vi "Car Wash.vi"() -> ()   [LabVIEW 2021]
doc: "car wash by Jeremy"
uses:
  Controls/Car Wash Indicators.ctl
  Controls/Wash Options.ctl
  Controls/states.ctl
panel:
  in  "Start":bool
  out "Elapsed Time":dbl format="%0.2f"
  in  "stop":bool
  out "Wash Entry":bool
  in  "Wash Options":T1
  in  "Car Position Slider":u8(slide) max=3 scale=0.0..4.0
  out "Car Wash Indicators":T2
  # "Entry Console"
  # "Car Wash Display"
  # "Car Position Simulation"
  # "Pre-Soak\nH-P Wash\nL-P Wax\nSpot Free Rinse"
  # "Underbody Wash\nBug Remover"
  # "Tire Shine\nAir Dry"
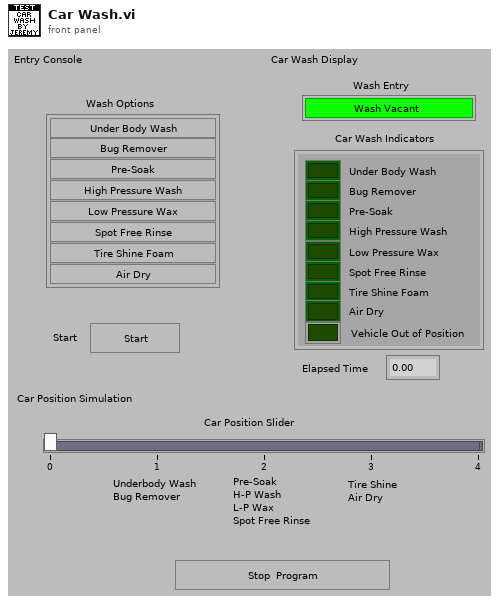
[diagram p1: front panel]
types:
  T1 = typedef "Wash Options.ctl" = cluster{"Underbody Wash":bool, "Bug Remover":bool, "Pre-Soak":bool, "High Pressure Wash":bool, "Low Pressure Wax":bool, "Spot Free Rinse":bool, "Tire Shine Foam":bool, "Air Dry":bool}
  T2 = typedef "Car Wash Indicators.ctl" = cluster{"Under Body Wash":bool, "Bug Remover":bool, "Pre-Soak":bool, "High Pressure Wash":bool, "Low Pressure Wax":bool, "Spot Free Rinse":bool, "Tire Shine Foam":bool, "Air Dry":bool, "Vehicle Out of Position":bool}
  T3 = typedef "states.ctl" = enum16{"Init", "Select Wash Options", "Configure Options", "Under Body Wash", "Bug Remover", "Pre-Soak", "High Pressure Wash", "Low Pressure Wax", "Spot Free Rinse", "Tire Shine Foam", "Air Dry", "Skip", "Exit", "Stop"}
  T4 = enum8{"Enabled", "Disabled", "Disabled and Grayed Out"}
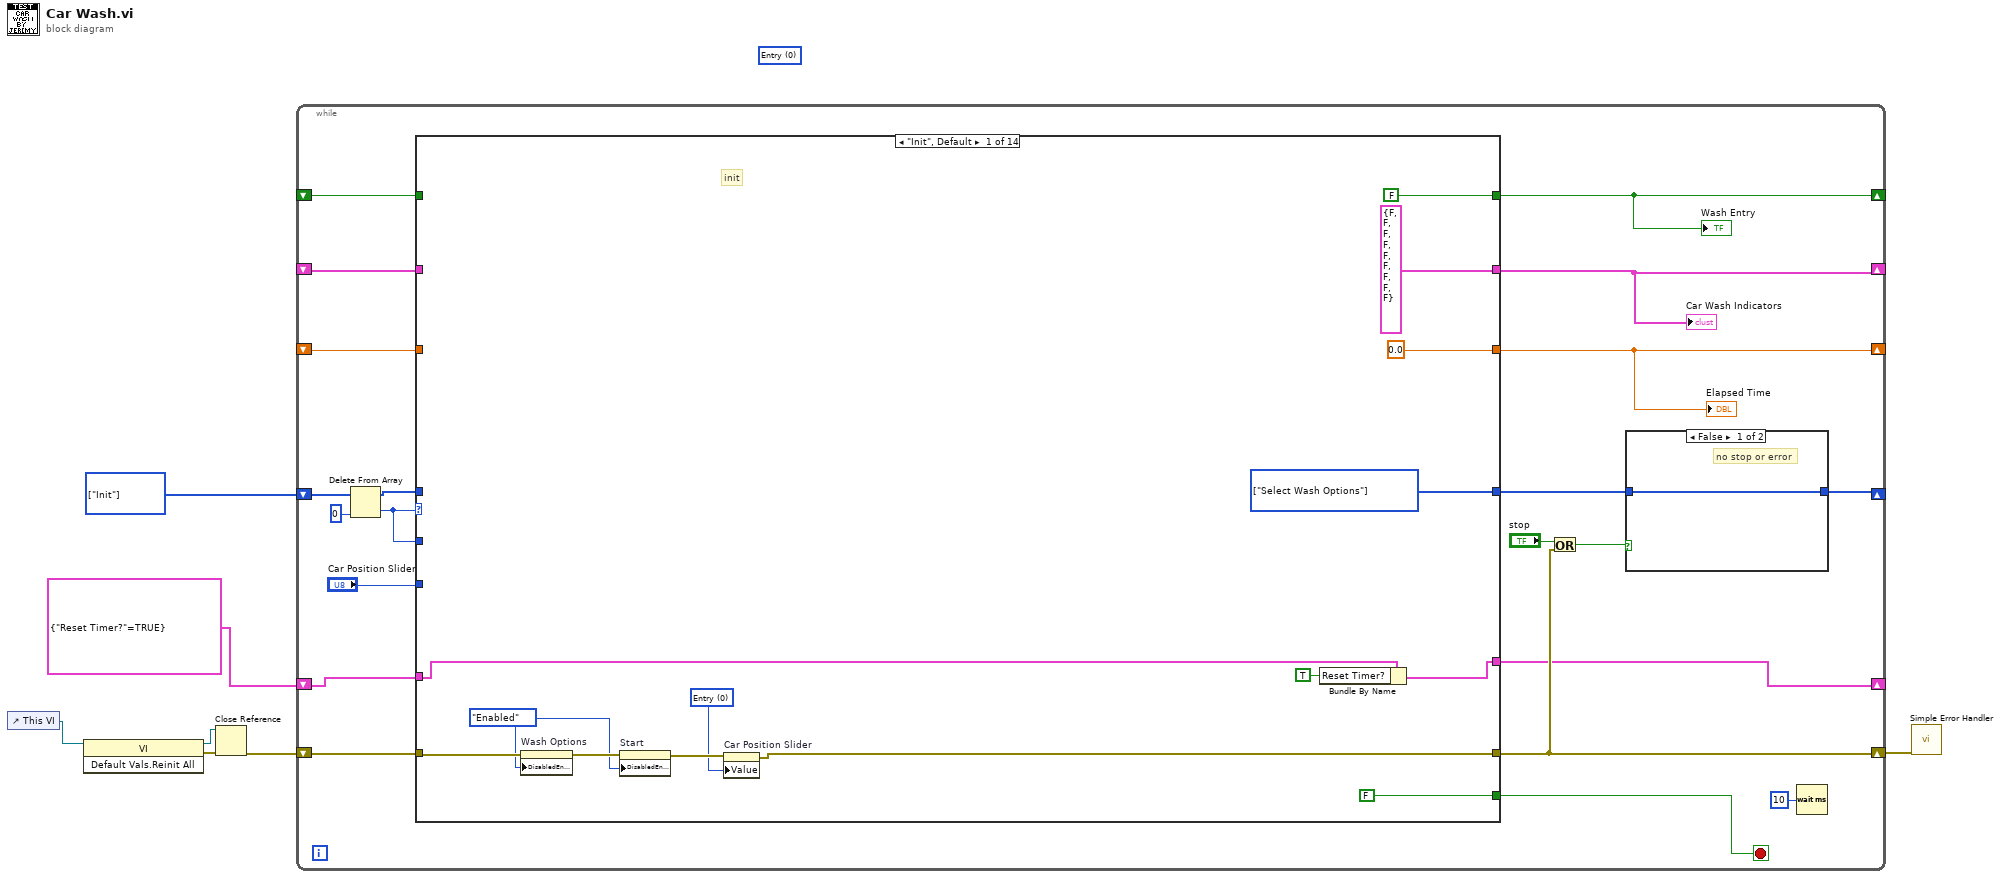
[diagram p0: block diagram]
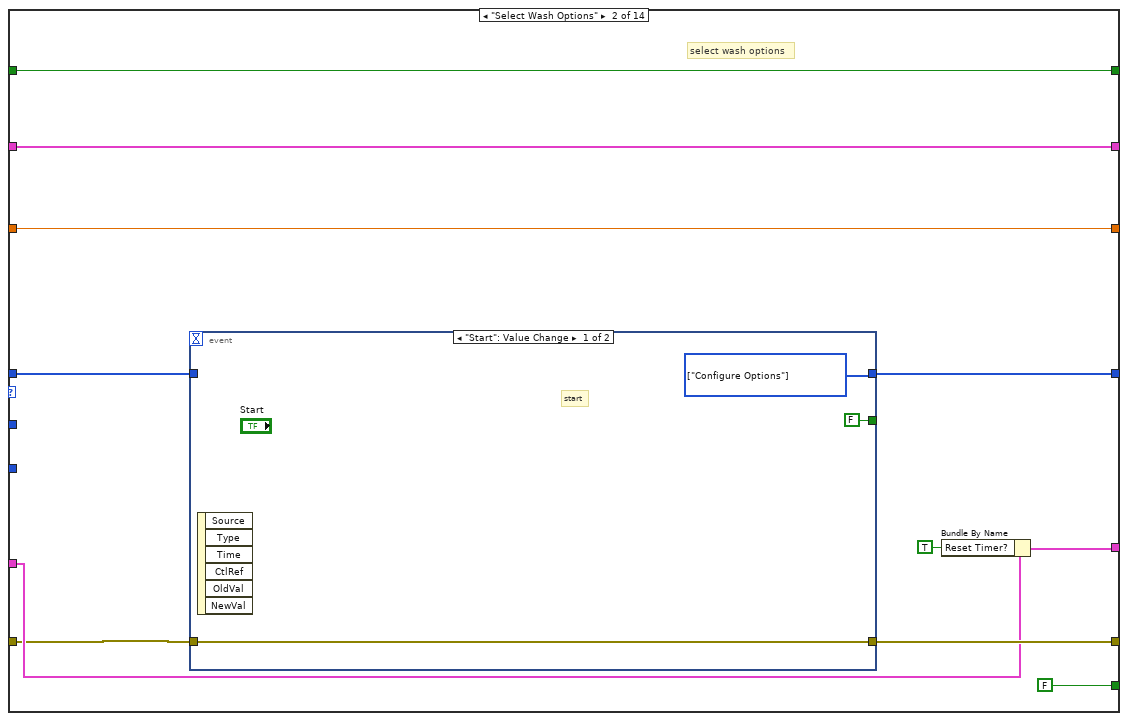
[diagram p2: hidden frame]
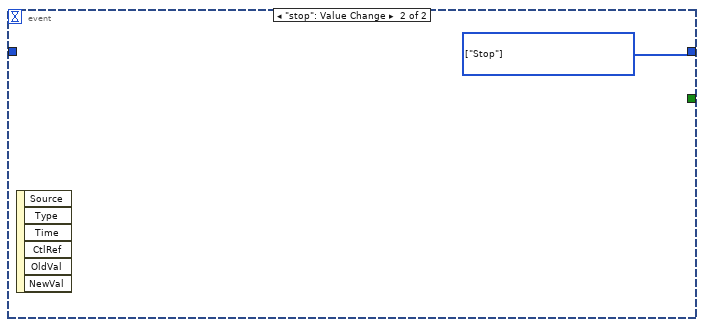
[diagram p3: hidden frame]
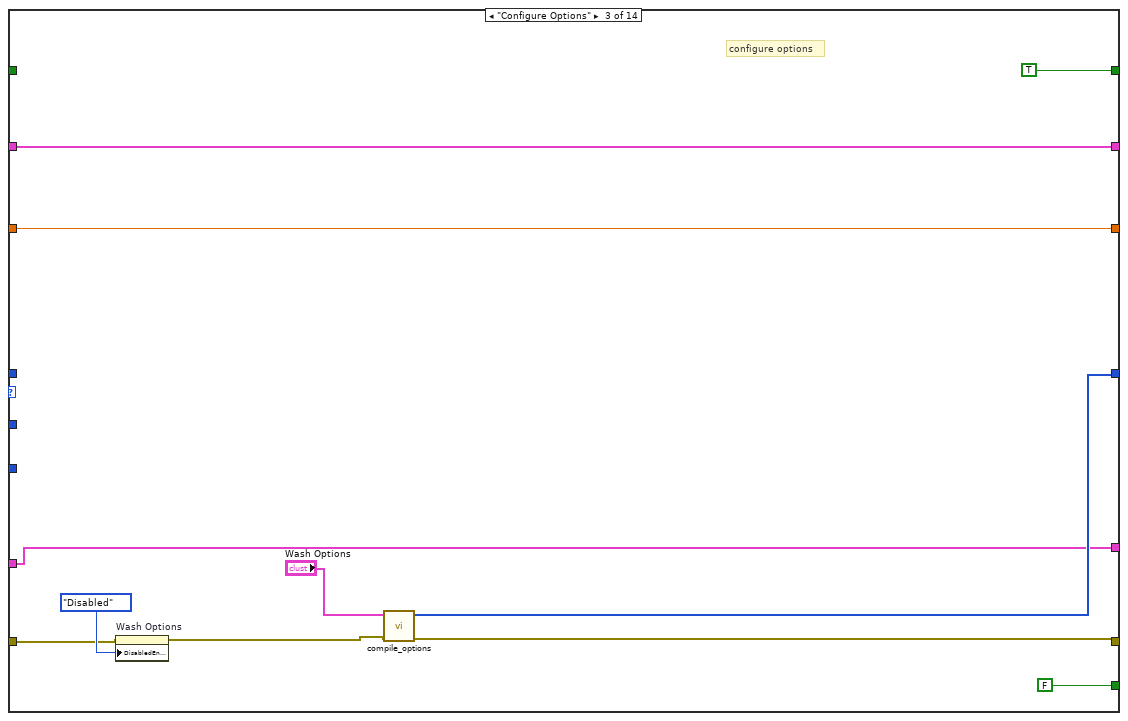
[diagram p4: hidden frame]
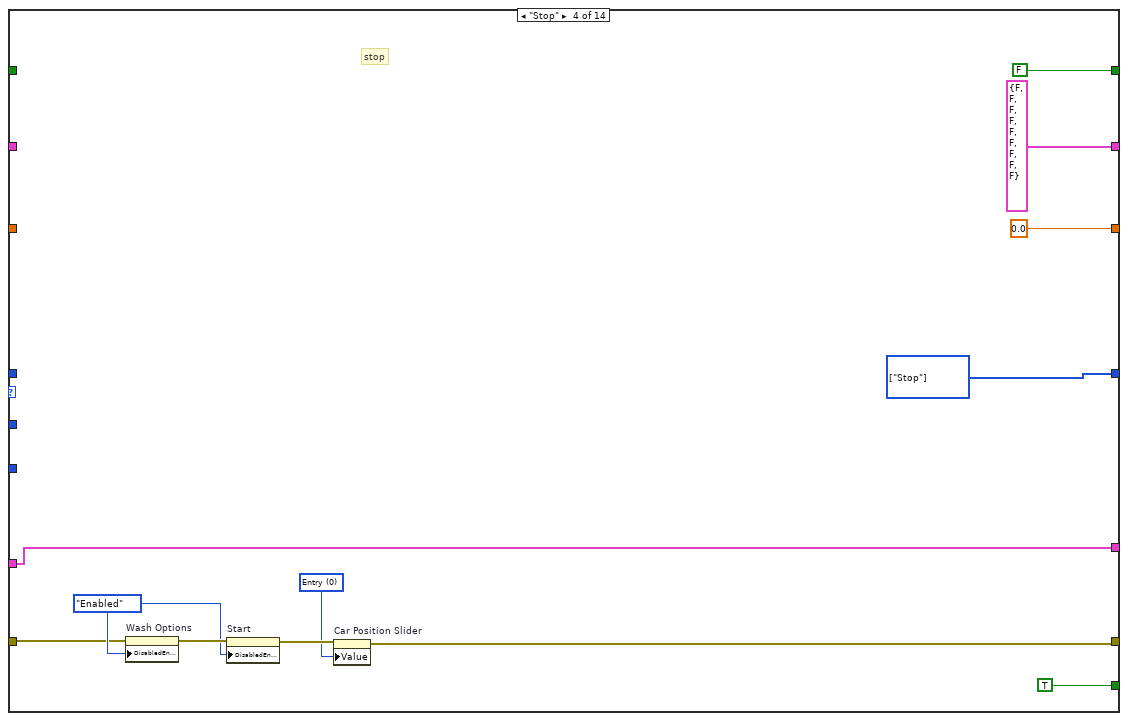
[diagram p5: hidden frame]
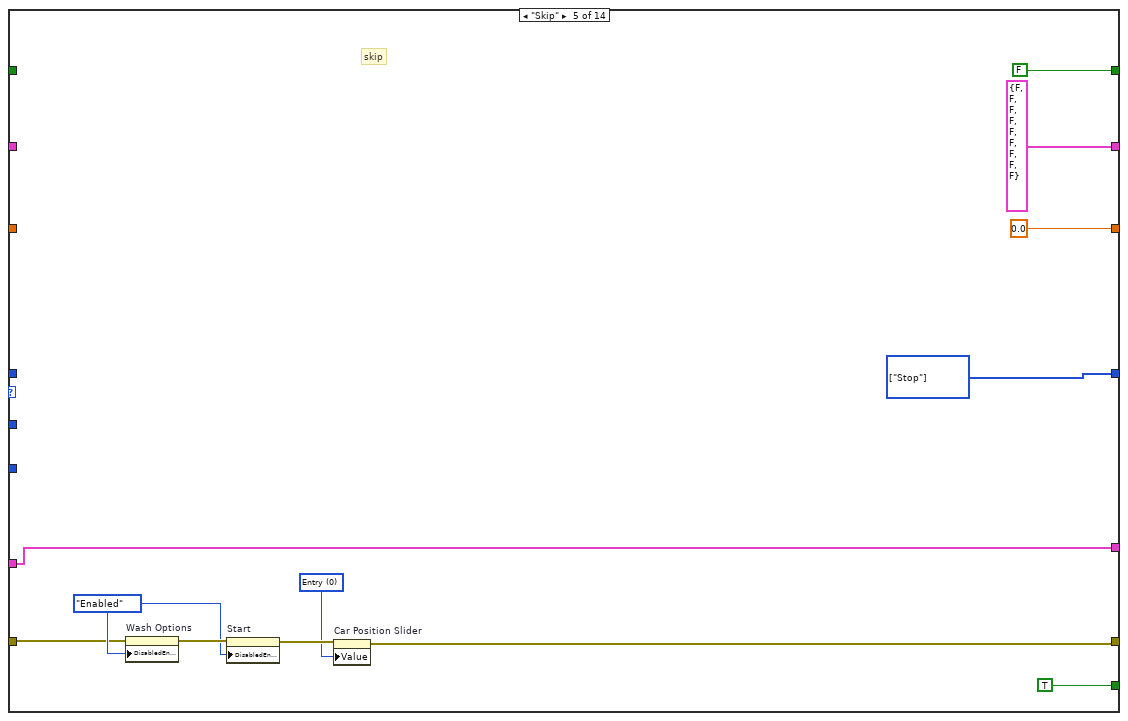
[diagram p6: hidden frame]
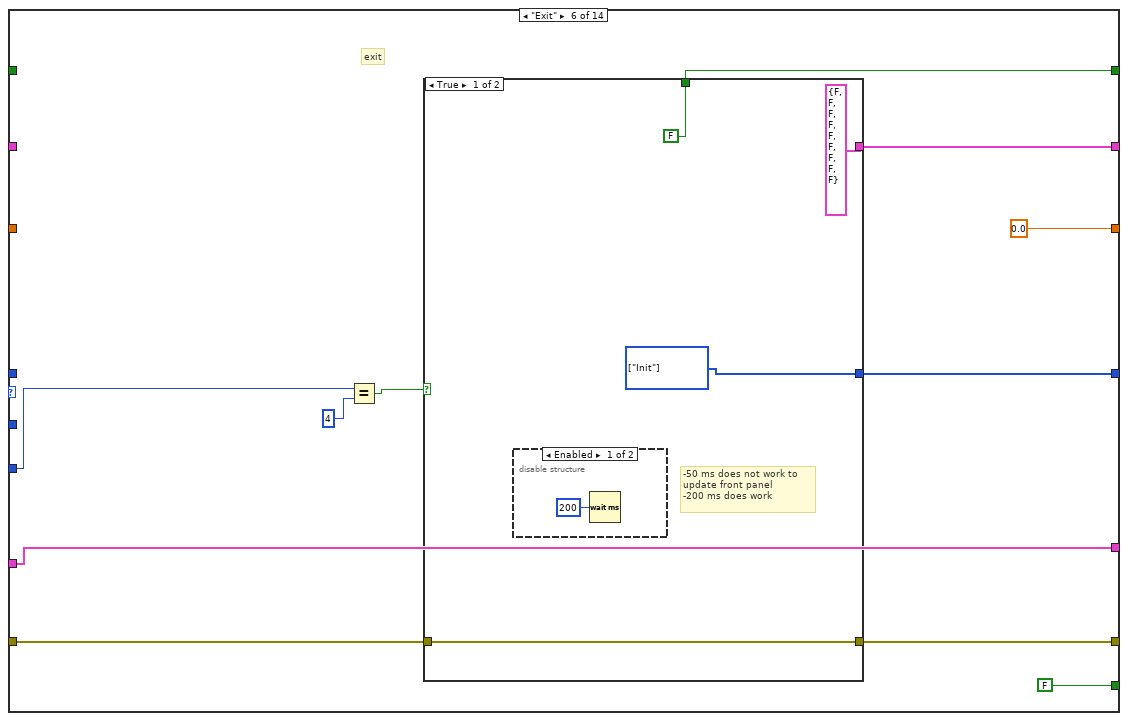
[diagram p7: hidden frame]
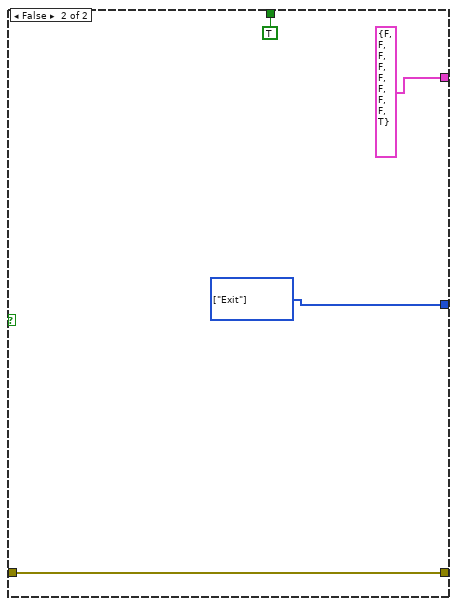
[diagram p9: hidden frame]
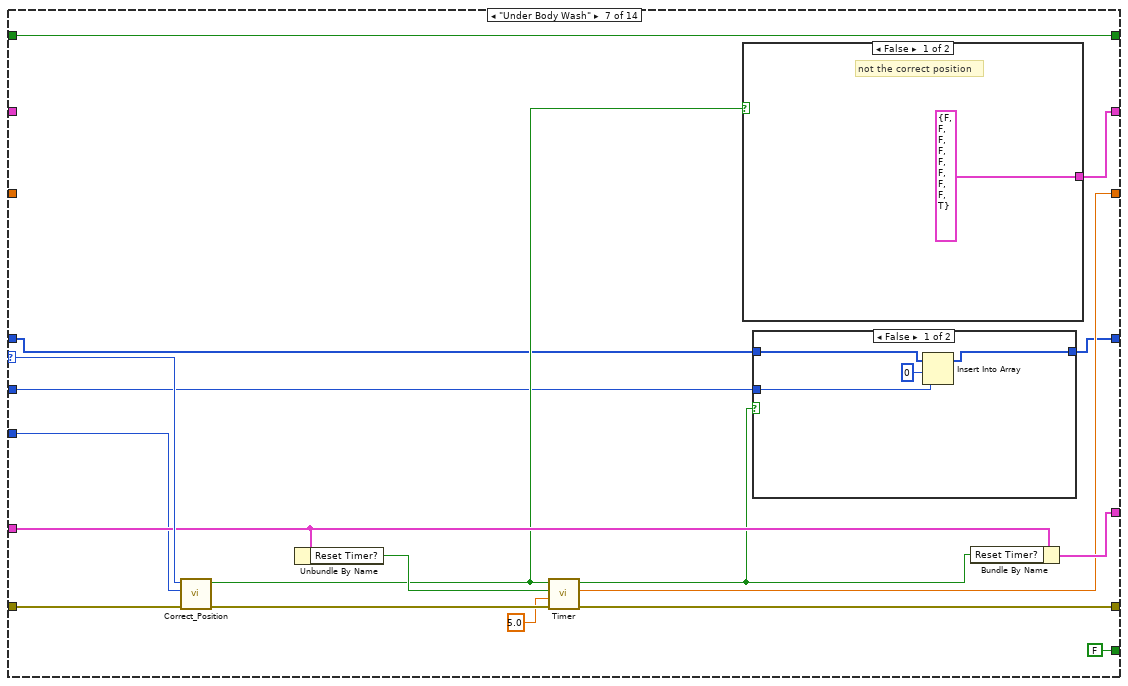
[diagram p10: hidden frame]
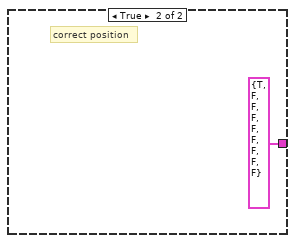
[diagram p12: hidden frame]
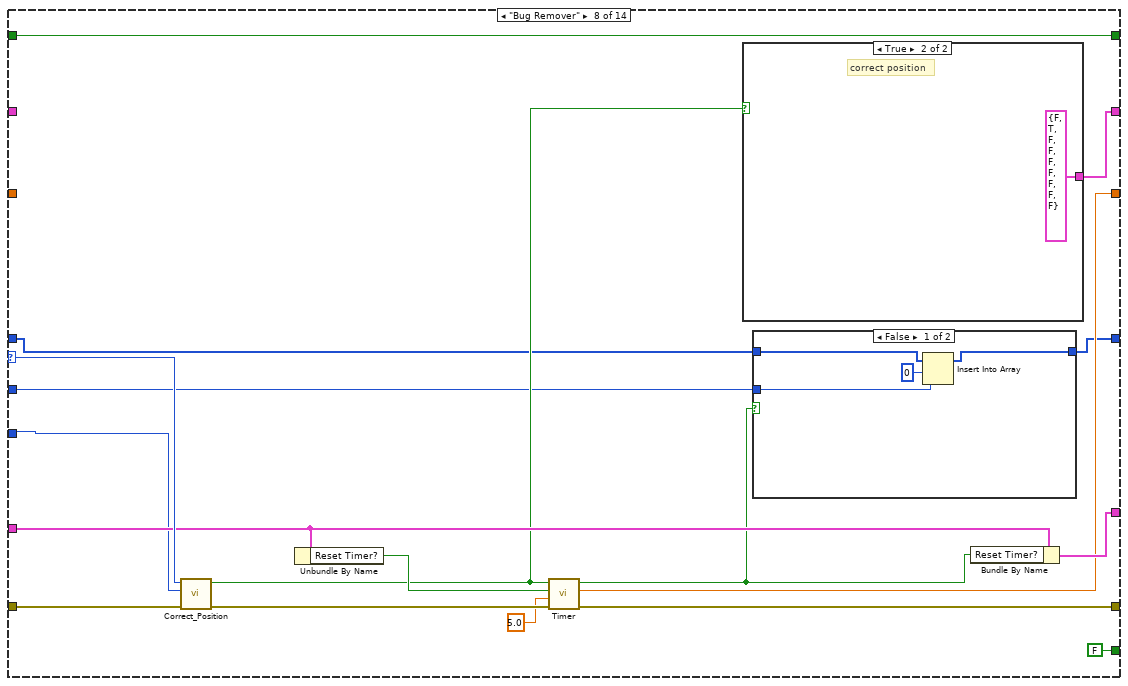
[diagram p13: hidden frame]
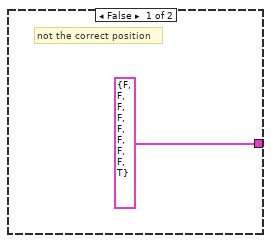
[diagram p15: hidden frame]
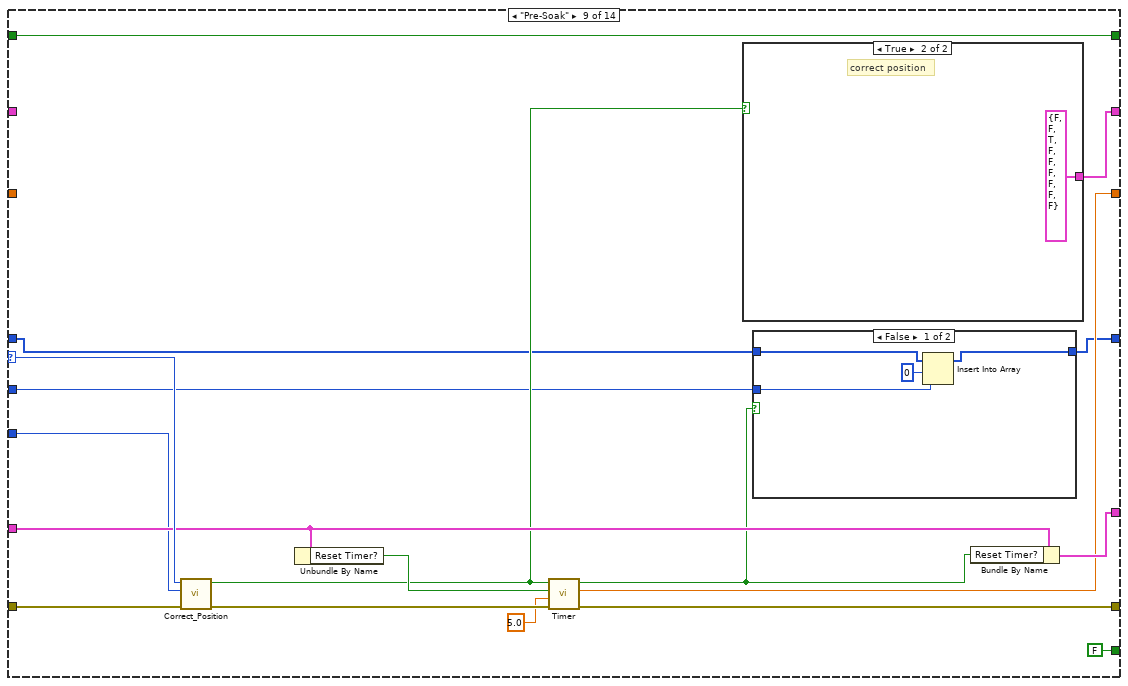
[diagram p16: hidden frame]
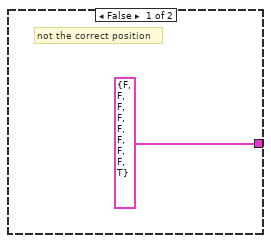
[diagram p18: hidden frame]
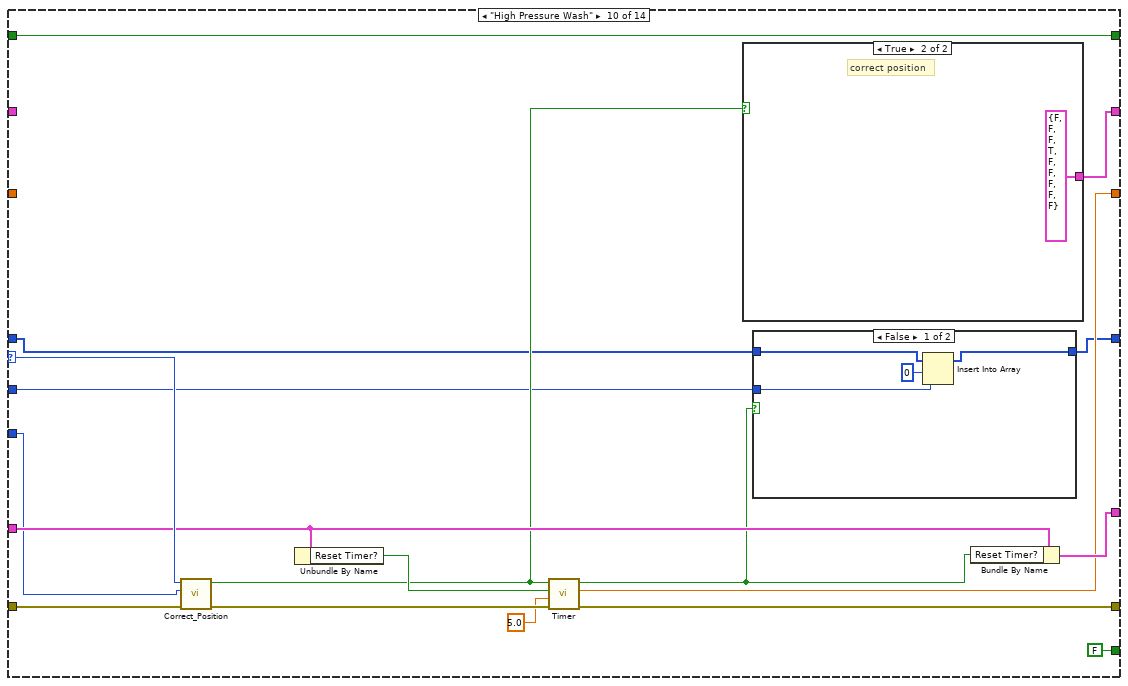
[diagram p19: hidden frame]
diagram:
  (unwired) u8 0 items=["Entry", "Station 1", "Station 2", "Station 3", "Exit"] ("Car Position Slider")
  w4 = T3[] [enum."Init"] items=["Init", "Select Wash Options", "Configure Options", "Under Body Wash", "Bug Remover", "Pre-Soak", "High Pressure Wash", "Low Pressure Wax", "Spot Free Rinse", "Tire Shine Foam", "Air Dry", "Skip", "Exit", "Stop"]
  n1 = control-ref of="This VI"() -> (w7:refnum<vi>)
  n2 = invoke class="VI" method="Default Vals.Reinit All"(reference=w7) -> (reference out=w5:refnum<vi>, error out=w6:errorcluster)  [unwired: 2 in, 1 out]
  n3 = Close Reference(reference=w5, error in (no error)=w6) -> (error out=w1:errorcluster)
  n4 = while {
    shift-right: [w17] -> w2
    shift-left: w1 -> [w9]
    shift-right: [w19] -> _
    shift-left: w4 -> [w28]
    shift-right: [w21] -> _
    shift-left: _ -> [w24]
    shift-right: [w20] -> _
    shift-left: _ -> [w25]
    shift-right: [w22] -> _
    shift-left: _ -> [w23]
    shift-right: [w13] -> _
    shift-left: cluster{"Reset Timer?":bool} {"Reset Timer?"=TRUE} -> [w14]
    stop <- w26 stop-if-true
    n5 = Delete From Array(array=w28, index=0) -> (deleted portion=w12:T3, array with subset deleted=w27:T3[])  [unwired: 1 in]
    n6 = case shown="\"Init\", Default" w12 {
      selector: w12 -> [_ _ _ _ _ _ w127 w152 w177 w203 w227 w253 w277 w302]
      tunnel: w9 -> [w42 w43 w64 w74 w86 w94 w130 w155 w180 w189 w230 w239 w280 w305]
      tunnel: [T2 {"Under Body Wash"=FALSE, "Bug Remover"=FALSE, "Pre-Soak"=FALSE, "High Pressure Wash"=FALSE, "Low Pressure Wax"=FALSE, "Spot Free Rinse"=FALSE, "Tire Shine Foam"=FALSE, "Air Dry"=FALSE, "Vehicle Out of Position"=FALSE} ("Car Wash Indicators") w50 w63 T2 {"Under Body Wash"=FALSE, "Bug Remover"=FALSE, "Pre-Soak"=FALSE, "High Pressure Wash"=FALSE, "Low Pressure Wax"=FALSE, "Spot Free Rinse"=FALSE, "Tire Shine Foam"=FALSE, "Air Dry"=FALSE, "Vehicle Out of Position"=FALSE} ("Car Wash Indicators") T2 {"Under Body Wash"=FALSE, "Bug Remover"=FALSE, "Pre-Soak"=FALSE, "High Pressure Wash"=FALSE, "Low Pressure Wax"=FALSE, "Spot Free Rinse"=FALSE, "Tire Shine Foam"=FALSE, "Air Dry"=FALSE, "Vehicle Out of Position"=FALSE} ("Car Wash Indicators") w97 w118 w143 w168 w194 w218 w244 w268 w293] -> w21
      tunnel: [0.0 ("Elapsed Time") w51 w68 0.0 ("Elapsed Time") 0.0 ("Elapsed Time") 0.0 ("Elapsed Time") w121 w146 w171 w197 w221 w247 w271 w296] -> w22
      tunnel: [FALSE ("Wash Entry") w49 TRUE ("Wash Entry") FALSE ("Wash Entry") FALSE ("Wash Entry") w96 w129 w154 w179 w205 w229 w255 w279 w304] -> w20
      tunnel: [w35 w53 w60 w70 w82 w95 w125 w150 w175 w201 w225 w251 w275 w300] -> w17
      tunnel: [w34 w47 w59 w79 w91 w100 w115 w140 w165 w191 w215 w241 w265 w290] -> w11
      tunnel: w27 -> [_ w52 _ _ _ _ w117 w142 w167 w193 w217 w243 w267 w292]
      tunnel: [FALSE FALSE FALSE TRUE TRUE FALSE FALSE FALSE FALSE FALSE FALSE FALSE FALSE FALSE] -> w26
      tunnel: w25 -> [_ w49 _ _ _ _ w129 w154 w179 w205 w229 w255 w279 w304]
      tunnel: w24 -> [_ w50 w63 _ _ _ _ _ _ _ _ _ _ _]
      tunnel: w23 -> [_ w51 w68 _ _ _ _ _ _ _ _ _ _ _]
      tunnel: [w31 w44 w58 w69 w81 w101 w122 w147 w172 w198 w222 w248 w272 w297] -> w13
      tunnel: w14 -> [w32 w45 w58 w69 w81 w101 w123 w148 w173 w199 w223 w249 w273 w298]
      tunnel: w12 -> [_ _ _ _ _ _ w114 w139 w164 w190 w214 w240 w264 w289]
      tunnel: "Car Position Slider" -> [_ _ _ _ _ w93 w113 w138 w163 w188 w213 w238 w263 w288]
      frame "Init", Default {
        w29 = u8 0 items=["Entry", "Station 1", "Station 2", "Station 3", "Exit"] ("Car Position Slider")
        w34 = T3[] [enum."Select Wash Options"] items=["Init", "Select Wash Options", "Configure Options", "Under Body Wash", "Bug Remover", "Pre-Soak", "High Pressure Wash", "Low Pressure Wax", "Spot Free Rinse", "Tire Shine Foam", "Air Dry", "Skip", "Exit", "Stop"]
        w40 = T4."Enabled" ("Disabled")
        # "init"
        n7 = property on="Wash Options" class="Clust (strict)"(error in=w42, "DisabledEnum"=w40) -> (error out=w41:errorcluster)  [unwired: 1 in, 1 out]
        n8 = property on="Start" class="Bool"(error in=w41, "DisabledEnum"=w40) -> (error out=w36:errorcluster)  [unwired: 1 in, 1 out]
        n9 = property on="Car Position Slider" class="Slide (strict)"(error in=w36, "Value"=w29) -> (error out=w35:errorcluster)  [unwired: 1 in, 1 out]
        n10 = Bundle By Name(cluster=w32, "Reset Timer?"=TRUE) -> (w31:cluster{"Reset Timer?":bool})
      }
      frame "Select Wash Options" {
        # "select wash options"
        n11 = event shown="[0] \"Start\": Value Change" {
          selector: _ -> [_ _]
          dyn-events: _ -> [_ _]
          timeout: _ -> [_ _]
          tunnel: [w56 _] -> w53
          tunnel: w43 -> [w56 _]
          tunnel: [FALSE ("stop") _] -> _
          tunnel: [w54 w57] -> w47
          tunnel: w52 -> [_ _]
          event "Start": Value Change {
            w54 = T3[] [enum."Configure Options"] items=["Init", "Select Wash Options", "Configure Options", "Under Body Wash", "Bug Remover", "Pre-Soak", "High Pressure Wash", "Low Pressure Wax", "Spot Free Rinse", "Tire Shine Foam", "Air Dry", "Skip", "Exit", "Stop"]
            # "start"
            n12 = event-data() -> ()  [unwired: 1 in, 6 out]
          }
          event "stop": Value Change {
            w57 = T3[] [enum."Stop"] items=["Init", "Select Wash Options", "Configure Options", "Under Body Wash", "Bug Remover", "Pre-Soak", "High Pressure Wash", "Low Pressure Wax", "Spot Free Rinse", "Tire Shine Foam", "Air Dry", "Skip", "Exit", "Stop"]
            n13 = event-data() -> ()  [unwired: 1 in, 6 out]
          }
        }
        n14 = Bundle By Name(cluster=w45, "Reset Timer?"=TRUE) -> (w44:cluster{"Reset Timer?":bool})
      }
      frame "Configure Options" {
        # "configure options"
        n15 = property on="Wash Options" class="Clust (strict)"(error in=w64, "DisabledEnum"=T4."Disabled" ("Disabled")) -> (error out=w61:errorcluster)  [unwired: 1 in, 1 out]
        n16 = call "compile_options.vi"("error in (no error)"=w61, "Wash Options"="Wash Options") -> ("error out"=w60:errorcluster, "Options Array"=w59:T3[])  [unwired: 8 in]
      }
      frame "Stop" {
        w76 = u8 0 items=["Entry", "Station 1", "Station 2", "Station 3", "Exit"] ("Car Position Slider")
        w75 = T4."Enabled" ("Disabled")
        w79 = T3[] [enum."Stop"] items=["Init", "Select Wash Options", "Configure Options", "Under Body Wash", "Bug Remover", "Pre-Soak", "High Pressure Wash", "Low Pressure Wax", "Spot Free Rinse", "Tire Shine Foam", "Air Dry", "Skip", "Exit", "Stop"]
        # "stop"
        n17 = property on="Wash Options" class="Clust (strict)"(error in=w74, "DisabledEnum"=w75) -> (error out=w78:errorcluster)  [unwired: 1 in, 1 out]
        n18 = property on="Start" class="Bool"(error in=w78, "DisabledEnum"=w75) -> (error out=w77:errorcluster)  [unwired: 1 in, 1 out]
        n19 = property on="Car Position Slider" class="Slide (strict)"(error in=w77, "Value"=w76) -> (error out=w70:errorcluster)  [unwired: 1 in, 1 out]
      }
      frame "Skip" {
        w88 = u8 0 items=["Entry", "Station 1", "Station 2", "Station 3", "Exit"] ("Car Position Slider")
        w87 = T4."Enabled" ("Disabled")
        w91 = T3[] [enum."Stop"] items=["Init", "Select Wash Options", "Configure Options", "Under Body Wash", "Bug Remover", "Pre-Soak", "High Pressure Wash", "Low Pressure Wax", "Spot Free Rinse", "Tire Shine Foam", "Air Dry", "Skip", "Exit", "Stop"]
        # "skip"
        n20 = property on="Wash Options" class="Clust (strict)"(error in=w86, "DisabledEnum"=w87) -> (error out=w90:errorcluster)  [unwired: 1 in, 1 out]
        n21 = property on="Start" class="Bool"(error in=w90, "DisabledEnum"=w87) -> (error out=w89:errorcluster)  [unwired: 1 in, 1 out]
        n22 = property on="Car Position Slider" class="Slide (strict)"(error in=w89, "Value"=w88) -> (error out=w82:errorcluster)  [unwired: 1 in, 1 out]
      }
      frame "Exit" {
        # "exit"
        n23 = Equal?(x=w93, y=u8 4) -> (x = y?=w99:bool)
        n24 = case shown="True" w99 {
          tunnel: [w107 w112] -> w100
          tunnel: [T2 {"Under Body Wash"=FALSE, "Bug Remover"=FALSE, "Pre-Soak"=FALSE, "High Pressure Wash"=FALSE, "Low Pressure Wax"=FALSE, "Spot Free Rinse"=FALSE, "Tire Shine Foam"=FALSE, "Air Dry"=FALSE, "Vehicle Out of Position"=FALSE} ("Car Wash Indicators") T2 {"Under Body Wash"=FALSE, "Bug Remover"=FALSE, "Pre-Soak"=FALSE, "High Pressure Wash"=FALSE, "Low Pressure Wax"=FALSE, "Spot Free Rinse"=FALSE, "Tire Shine Foam"=FALSE, "Air Dry"=FALSE, "Vehicle Out of Position"=TRUE} ("Car Wash Indicators")] -> w97
          tunnel: w94 -> [w104 w109]
          tunnel: [FALSE ("Wash Entry") TRUE ("Wash Entry")] -> w96
          tunnel: [w104 w109] -> w95
          frame True {
            w107 = T3[] [enum."Init"] items=["Init", "Select Wash Options", "Configure Options", "Under Body Wash", "Bug Remover", "Pre-Soak", "High Pressure Wash", "Low Pressure Wax", "Spot Free Rinse", "Tire Shine Foam", "Air Dry", "Skip", "Exit", "Stop"]
            # "-50 ms does not work to \nupdate front panel\n-200 ms does work"
            n25 = disable-structure shown="Enabled" {
              frame Enabled {
                n26 = Wait (ms)(milliseconds to wait=u32 200) -> ()  [unwired: 1 out]
              }
              frame Disabled {
              }
            }
          }
          frame False {
            w112 = T3[] [enum."Exit"] items=["Init", "Select Wash Options", "Configure Options", "Under Body Wash", "Bug Remover", "Pre-Soak", "High Pressure Wash", "Low Pressure Wax", "Spot Free Rinse", "Tire Shine Foam", "Air Dry", "Skip", "Exit", "Stop"]
          }
        }
      }
      frame "Under Body Wash" {
        n27 = call "Correct_Position.vi"("error in (no error)"=w130, "Car Position Slider"=w113, "Enum"=w127) -> ("error out"=w126:errorcluster, "In Correct Position?"=w119:bool)  [unwired: 7 in]
        n28 = Unbundle By Name(w123) -> ("Reset Timer?"=w124:bool)
        n29 = call "Timer.vi"("error in (no error)"=w126, "Time Limit"=5.0, "Reset?"=w124, "Advance Time?"=w119) -> ("error out"=w125:errorcluster, "Time Elapsed"=w121:dbl, "Time Expired?"=w116:bool)  [unwired: 5 in]
        n30 = case shown="False" w119 {
          tunnel: [T2 {"Under Body Wash"=FALSE, "Bug Remover"=FALSE, "Pre-Soak"=FALSE, "High Pressure Wash"=FALSE, "Low Pressure Wax"=FALSE, "Spot Free Rinse"=FALSE, "Tire Shine Foam"=FALSE, "Air Dry"=FALSE, "Vehicle Out of Position"=TRUE} ("Car Wash Indicators") T2 {"Under Body Wash"=TRUE, "Bug Remover"=FALSE, "Pre-Soak"=FALSE, "High Pressure Wash"=FALSE, "Low Pressure Wax"=FALSE, "Spot Free Rinse"=FALSE, "Tire Shine Foam"=FALSE, "Air Dry"=FALSE, "Vehicle Out of Position"=FALSE} ("Car Wash Indicators")] -> w118
          frame False {
            # "not the correct position"
          }
          frame True {
            # "correct position"
          }
        }
        n31 = case shown="False" w116 {
          tunnel: w117 -> [w134 w135]
          tunnel: [w131 w135] -> w115
          tunnel: w114 -> [w132 _]
          frame False {
            n32 = Insert Into Array(array=w134, index=0, new element=w132) -> (w131:T3[])
          }
          frame True {
            # "time expired.  Case done"
          }
        }
        n33 = Bundle By Name(cluster=w123, "Reset Timer?"=w116) -> (w122:cluster{"Reset Timer?":bool})
      }
      frame "Bug Remover" {
        n34 = call "Correct_Position.vi"("error in (no error)"=w155, "Car Position Slider"=w138, "Enum"=w152) -> ("error out"=w151:errorcluster, "In Correct Position?"=w144:bool)  [unwired: 7 in]
        n35 = Unbundle By Name(w148) -> ("Reset Timer?"=w149:bool)
        n36 = call "Timer.vi"("error in (no error)"=w151, "Time Limit"=5.0, "Reset?"=w149, "Advance Time?"=w144) -> ("error out"=w150:errorcluster, "Time Elapsed"=w146:dbl, "Time Expired?"=w141:bool)  [unwired: 5 in]
        n37 = case shown="True" w144 {
          tunnel: [T2 {"Under Body Wash"=FALSE, "Bug Remover"=FALSE, "Pre-Soak"=FALSE, "High Pressure Wash"=FALSE, "Low Pressure Wax"=FALSE, "Spot Free Rinse"=FALSE, "Tire Shine Foam"=FALSE, "Air Dry"=FALSE, "Vehicle Out of Position"=TRUE} ("Car Wash Indicators") T2 {"Under Body Wash"=FALSE, "Bug Remover"=TRUE, "Pre-Soak"=FALSE, "High Pressure Wash"=FALSE, "Low Pressure Wax"=FALSE, "Spot Free Rinse"=FALSE, "Tire Shine Foam"=FALSE, "Air Dry"=FALSE, "Vehicle Out of Position"=FALSE} ("Car Wash Indicators")] -> w143
          frame False {
            # "not the correct position"
          }
          frame True {
            # "correct position"
          }
        }
        n38 = case shown="False" w141 {
          tunnel: w142 -> [w159 w160]
          tunnel: [w156 w160] -> w140
          tunnel: w139 -> [w157 _]
          frame False {
            n39 = Insert Into Array(array=w159, index=0, new element=w157) -> (w156:T3[])
          }
          frame True {
            # "time expired.  Case done"
          }
        }
        n40 = Bundle By Name(cluster=w148, "Reset Timer?"=w141) -> (w147:cluster{"Reset Timer?":bool})
      }
      frame "Pre-Soak" {
        n41 = call "Correct_Position.vi"("error in (no error)"=w180, "Car Position Slider"=w163, "Enum"=w177) -> ("error out"=w176:errorcluster, "In Correct Position?"=w169:bool)  [unwired: 7 in]
        n42 = Unbundle By Name(w173) -> ("Reset Timer?"=w174:bool)
        n43 = call "Timer.vi"("error in (no error)"=w176, "Time Limit"=5.0, "Reset?"=w174, "Advance Time?"=w169) -> ("error out"=w175:errorcluster, "Time Elapsed"=w171:dbl, "Time Expired?"=w166:bool)  [unwired: 5 in]
        n44 = case shown="True" w169 {
          tunnel: [T2 {"Under Body Wash"=FALSE, "Bug Remover"=FALSE, "Pre-Soak"=FALSE, "High Pressure Wash"=FALSE, "Low Pressure Wax"=FALSE, "Spot Free Rinse"=FALSE, "Tire Shine Foam"=FALSE, "Air Dry"=FALSE, "Vehicle Out of Position"=TRUE} ("Car Wash Indicators") T2 {"Under Body Wash"=FALSE, "Bug Remover"=FALSE, "Pre-Soak"=TRUE, "High Pressure Wash"=FALSE, "Low Pressure Wax"=FALSE, "Spot Free Rinse"=FALSE, "Tire Shine Foam"=FALSE, "Air Dry"=FALSE, "Vehicle Out of Position"=FALSE} ("Car Wash Indicators")] -> w168
          frame False {
            # "not the correct position"
          }
          frame True {
            # "correct position"
          }
        }
        n45 = case shown="False" w166 {
          tunnel: w167 -> [w184 w185]
          tunnel: [w181 w185] -> w165
          tunnel: w164 -> [w182 _]
          frame False {
            n46 = Insert Into Array(array=w184, index=0, new element=w182) -> (w181:T3[])
          }
          frame True {
            # "time expired.  Case done"
          }
        }
        n47 = Bundle By Name(cluster=w173, "Reset Timer?"=w166) -> (w172:cluster{"Reset Timer?":bool})
      }
      frame "High Pressure Wash" {
        n48 = call "Correct_Position.vi"("error in (no error)"=w189, "Car Position Slider"=w188, "Enum"=w203) -> ("error out"=w202:errorcluster, "In Correct Position?"=w195:bool)  [unwired: 7 in]
        n49 = Unbundle By Name(w199) -> ("Reset Timer?"=w200:bool)
        n50 = call "Timer.vi"("error in (no error)"=w202, "Time Limit"=5.0, "Reset?"=w200, "Advance Time?"=w195) -> ("error out"=w201:errorcluster, "Time Elapsed"=w197:dbl, "Time Expired?"=w192:bool)  [unwired: 5 in]
        n51 = case shown="True" w195 {
          tunnel: [T2 {"Under Body Wash"=FALSE, "Bug Remover"=FALSE, "Pre-Soak"=FALSE, "High Pressure Wash"=FALSE, "Low Pressure Wax"=FALSE, "Spot Free Rinse"=FALSE, "Tire Shine Foam"=FALSE, "Air Dry"=FALSE, "Vehicle Out of Position"=TRUE} ("Car Wash Indicators") T2 {"Under Body Wash"=FALSE, "Bug Remover"=FALSE, "Pre-Soak"=FALSE, "High Pressure Wash"=TRUE, "Low Pressure Wax"=FALSE, "Spot Free Rinse"=FALSE, "Tire Shine Foam"=FALSE, "Air Dry"=FALSE, "Vehicle Out of Position"=FALSE} ("Car Wash Indicators")] -> w194
          frame False {
            # "not the correct position"
          }
          frame True {
            # "correct position"
          }
        }
        n52 = case shown="False" w192 {
          tunnel: w193 -> [w209 w210]
          tunnel: [w206 w210] -> w191
          tunnel: w190 -> [w207 _]
          frame False {
            n53 = Insert Into Array(array=w209, index=0, new element=w207) -> (w206:T3[])
          }
          frame True {
            # "time expired.  Case done"
          }
        }
        n54 = Bundle By Name(cluster=w199, "Reset Timer?"=w192) -> (w198:cluster{"Reset Timer?":bool})
      }
      frame "Low Pressure Wax" {
        n55 = call "Correct_Position.vi"("error in (no error)"=w230, "Car Position Slider"=w213, "Enum"=w227) -> ("error out"=w226:errorcluster, "In Correct Position?"=w219:bool)  [unwired: 7 in]
        n56 = Unbundle By Name(w223) -> ("Reset Timer?"=w224:bool)
        n57 = call "Timer.vi"("error in (no error)"=w226, "Time Limit"=5.0, "Reset?"=w224, "Advance Time?"=w219) -> ("error out"=w225:errorcluster, "Time Elapsed"=w221:dbl, "Time Expired?"=w216:bool)  [unwired: 5 in]
        n58 = case shown="True" w219 {
          tunnel: [T2 {"Under Body Wash"=FALSE, "Bug Remover"=FALSE, "Pre-Soak"=FALSE, "High Pressure Wash"=FALSE, "Low Pressure Wax"=FALSE, "Spot Free Rinse"=FALSE, "Tire Shine Foam"=FALSE, "Air Dry"=FALSE, "Vehicle Out of Position"=TRUE} ("Car Wash Indicators") T2 {"Under Body Wash"=FALSE, "Bug Remover"=FALSE, "Pre-Soak"=FALSE, "High Pressure Wash"=FALSE, "Low Pressure Wax"=TRUE, "Spot Free Rinse"=FALSE, "Tire Shine Foam"=FALSE, "Air Dry"=FALSE, "Vehicle Out of Position"=FALSE} ("Car Wash Indicators")] -> w218
          frame False {
            # "not the correct position"
          }
          frame True {
            # "correct position"
          }
        }
        n59 = case shown="False" w216 {
          tunnel: w217 -> [w234 w235]
          tunnel: [w231 w235] -> w215
          tunnel: w214 -> [w232 _]
          frame False {
            n60 = Insert Into Array(array=w234, index=0, new element=w232) -> (w231:T3[])
          }
          frame True {
            # "time expired.  Case done"
          }
        }
        n61 = Bundle By Name(cluster=w223, "Reset Timer?"=w216) -> (w222:cluster{"Reset Timer?":bool})
      }
      frame "Spot Free Rinse" {
        n62 = call "Correct_Position.vi"("error in (no error)"=w239, "Car Position Slider"=w238, "Enum"=w253) -> ("error out"=w252:errorcluster, "In Correct Position?"=w245:bool)  [unwired: 7 in]
        n63 = Unbundle By Name(w249) -> ("Reset Timer?"=w250:bool)
        n64 = call "Timer.vi"("error in (no error)"=w252, "Time Limit"=5.0, "Reset?"=w250, "Advance Time?"=w245) -> ("error out"=w251:errorcluster, "Time Elapsed"=w247:dbl, "Time Expired?"=w242:bool)  [unwired: 5 in]
        n65 = case shown="True" w245 {
          tunnel: [T2 {"Under Body Wash"=FALSE, "Bug Remover"=FALSE, "Pre-Soak"=FALSE, "High Pressure Wash"=FALSE, "Low Pressure Wax"=FALSE, "Spot Free Rinse"=FALSE, "Tire Shine Foam"=FALSE, "Air Dry"=FALSE, "Vehicle Out of Position"=TRUE} ("Car Wash Indicators") T2 {"Under Body Wash"=FALSE, "Bug Remover"=FALSE, "Pre-Soak"=FALSE, "High Pressure Wash"=FALSE, "Low Pressure Wax"=FALSE, "Spot Free Rinse"=TRUE, "Tire Shine Foam"=FALSE, "Air Dry"=FALSE, "Vehicle Out of Position"=FALSE} ("Car Wash Indicators")] -> w244
          frame False {
            # "not the correct position"
          }
          frame True {
            # "correct position"
          }
        }
        n66 = case shown="False" w242 {
          tunnel: w243 -> [w259 w260]
          tunnel: [w256 w260] -> w241
          tunnel: w240 -> [w257 _]
          frame False {
            n67 = Insert Into Array(array=w259, index=0, new element=w257) -> (w256:T3[])
          }
          frame True {
            # "time expired.  Case done"
          }
        }
        n68 = Bundle By Name(cluster=w249, "Reset Timer?"=w242) -> (w248:cluster{"Reset Timer?":bool})
      }
      frame "Tire Shine Foam" {
        n69 = call "Correct_Position.vi"("error in (no error)"=w280, "Car Position Slider"=w263, "Enum"=w277) -> ("error out"=w276:errorcluster, "In Correct Position?"=w269:bool)  [unwired: 7 in]
        n70 = Unbundle By Name(w273) -> ("Reset Timer?"=w274:bool)
        n71 = call "Timer.vi"("error in (no error)"=w276, "Time Limit"=5.0, "Reset?"=w274, "Advance Time?"=w269) -> ("error out"=w275:errorcluster, "Time Elapsed"=w271:dbl, "Time Expired?"=w266:bool)  [unwired: 5 in]
        n72 = case shown="True" w269 {
          tunnel: [T2 {"Under Body Wash"=FALSE, "Bug Remover"=FALSE, "Pre-Soak"=FALSE, "High Pressure Wash"=FALSE, "Low Pressure Wax"=FALSE, "Spot Free Rinse"=FALSE, "Tire Shine Foam"=FALSE, "Air Dry"=FALSE, "Vehicle Out of Position"=TRUE} ("Car Wash Indicators") T2 {"Under Body Wash"=FALSE, "Bug Remover"=FALSE, "Pre-Soak"=FALSE, "High Pressure Wash"=FALSE, "Low Pressure Wax"=FALSE, "Spot Free Rinse"=FALSE, "Tire Shine Foam"=TRUE, "Air Dry"=FALSE, "Vehicle Out of Position"=FALSE} ("Car Wash Indicators")] -> w268
          frame False {
            # "not the correct position"
          }
          frame True {
            # "correct position"
          }
        }
        n73 = case shown="False" w266 {
          tunnel: w267 -> [w284 w285]
          tunnel: [w281 w285] -> w265
          tunnel: w264 -> [w282 _]
          frame False {
            n74 = Insert Into Array(array=w284, index=0, new element=w282) -> (w281:T3[])
          }
          frame True {
            # "time expired.  Case done"
          }
        }
        n75 = Bundle By Name(cluster=w273, "Reset Timer?"=w266) -> (w272:cluster{"Reset Timer?":bool})
      }
      frame "Air Dry" {
        n76 = call "Correct_Position.vi"("error in (no error)"=w305, "Car Position Slider"=w288, "Enum"=w302) -> ("error out"=w301:errorcluster, "In Correct Position?"=w294:bool)  [unwired: 7 in]
        n77 = Unbundle By Name(w298) -> ("Reset Timer?"=w299:bool)
        n78 = call "Timer.vi"("error in (no error)"=w301, "Time Limit"=5.0, "Reset?"=w299, "Advance Time?"=w294) -> ("error out"=w300:errorcluster, "Time Elapsed"=w296:dbl, "Time Expired?"=w291:bool)  [unwired: 5 in]
        n79 = case shown="True" w294 {
          tunnel: [T2 {"Under Body Wash"=FALSE, "Bug Remover"=FALSE, "Pre-Soak"=FALSE, "High Pressure Wash"=FALSE, "Low Pressure Wax"=FALSE, "Spot Free Rinse"=FALSE, "Tire Shine Foam"=FALSE, "Air Dry"=FALSE, "Vehicle Out of Position"=TRUE} ("Car Wash Indicators") T2 {"Under Body Wash"=FALSE, "Bug Remover"=FALSE, "Pre-Soak"=FALSE, "High Pressure Wash"=FALSE, "Low Pressure Wax"=FALSE, "Spot Free Rinse"=FALSE, "Tire Shine Foam"=FALSE, "Air Dry"=TRUE, "Vehicle Out of Position"=FALSE} ("Car Wash Indicators")] -> w293
          frame False {
            # "not the correct position"
          }
          frame True {
            # "correct position"
          }
        }
        n80 = case shown="False" w291 {
          tunnel: w292 -> [w309 w310]
          tunnel: [w306 w310] -> w290
          tunnel: w289 -> [w307 _]
          frame False {
            n81 = Insert Into Array(array=w309, index=0, new element=w307) -> (w306:T3[])
          }
          frame True {
            # "time expired.  Case done"
          }
        }
        n82 = Bundle By Name(cluster=w298, "Reset Timer?"=w291) -> (w297:cluster{"Reset Timer?":bool})
      }
    }
    "Elapsed Time" <- w22
    "Car Wash Indicators" <- w21
    "Wash Entry" <- w20
    n83 = Or(x="stop", y=w17) -> (x .or. y?=w16:bool)
    n84 = case shown="False" w16 {
      tunnel: [w313 w314] -> w19
      tunnel: w11 -> [w313 _]
      frame False {
        # "no stop or error"
      }
      frame True {
        w314 = T3[] [enum."Stop"] items=["Init", "Select Wash Options", "Configure Options", "Under Body Wash", "Bug Remover", "Pre-Soak", "High Pressure Wash", "Low Pressure Wax", "Spot Free Rinse", "Tire Shine Foam", "Air Dry", "Skip", "Exit", "Stop"]
        # "stop or error"
      }
    }
    n85 = Wait (ms)(milliseconds to wait=u32 10) -> ()  [unwired: 1 out]
  }
  n86 = call <vilib>:"Simple Error Handler.vi"("error in (no error)"=w2) -> ()  [unwired: 4 in, 5 out]
